vi "Opposite Edge.vi"(11 "edge in":enum16{"rising", "falling"}(ring)) -> (3 "opposite edge out":enum16{"rising", "falling"}(ring))   [LabVIEW 2013, in "I2S-TDM.lvlib"]
uses:
  I2S-TDM.lvlib
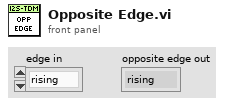
[diagram p1: front panel]
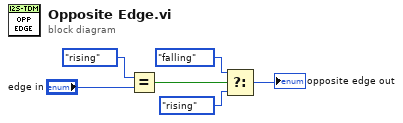
[diagram p0: block diagram]
diagram:
  n1 = Equal?(x=enum16{"rising", "falling"}."rising" ("edge (rising)"), y="edge in") -> (x = y?=w3:bool)
  n2 = Select(t=enum16{"rising", "falling"}."falling" ("edge (rising)"), s=w3, f=enum16{"rising", "falling"}."rising" ("edge (rising)")) -> (s? t:f=→"opposite edge out":enum16{"rising", "falling"})
